vi "Frame Load Bmp and Img.vi"(8 "error in (no error)":errorcluster, 9 "PNG Path":path, 10 "File String":string, 11 "LF2R IDE in":refnum<class "LF2R IDE.lvclass">) -> (0 "error out":errorcluster, 3 "LF2R IDE out":refnum<class "LF2R IDE.lvclass">)   [LabVIEW 2018, in "LF2R IDE.lvlib" / "LF2R IDE.lvclass"]
uses:
  LF2R IDE.lvclass
  LF2R IDE.lvclass/LF2R IDE.ctl
  Frame Analizer/Data Parser.lvclass
  Image/Image Process.lvclass
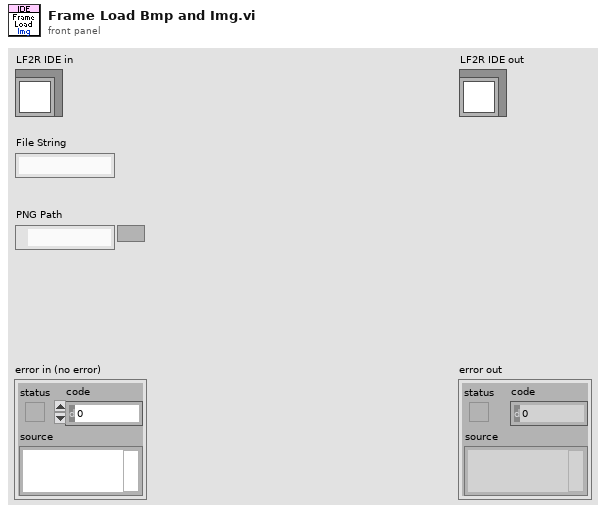
[diagram p1: front panel]
types:
  T1 = typedef "Data Parser.lvclass/Bmp data.ctl" = cluster{"File Data":T2[], "resized":string, "default_centerx":string, "default_centery":string}
  T2 = typedef "Data Parser.lvclass/Bmp File Data.ctl" = cluster{"Pic Start":i32, "Pic End":i32, "Json Path":string, "w":i32, "h":i32, "row":i32, "col":i32}
  T3 = typedef "Image Json Parser.lvclass/Img Json Data.ctl" = cluster{"frames":T4[], "meta":T5}
  T4 = typedef "Image Json Parser.lvclass/Img Json Frames.ctl" = cluster{"frame":cluster{"x":i32, "y":i32, "w":i32, "h":i32}, "rotated":bool, "trimmed":bool, "spriteSourceSize":cluster{"x":i32, "y":i32, "w":i32, "h":i32}, "sourceSize":cluster{"w":i32, "h":i32}}
  T5 = typedef "Image Json Parser.lvclass/Img Json Meta.ctl" = cluster{"app":string, "version":string, "image":string, "format":string, "size":cluster{"w":i32, "h":i32}, "scale":string}
  T6 = typedef "imagedata.ctl" = cluster{"image type":i32, "image depth":i32, "image":u8[], "mask":u8[], "colors":u32[], "Rectangle":cluster{"left":i16, "top":i16, "right":i16, "bottom":i16}}
  T7 = cluster{"image data":T6, "24-bit pixmap":u32[][]}
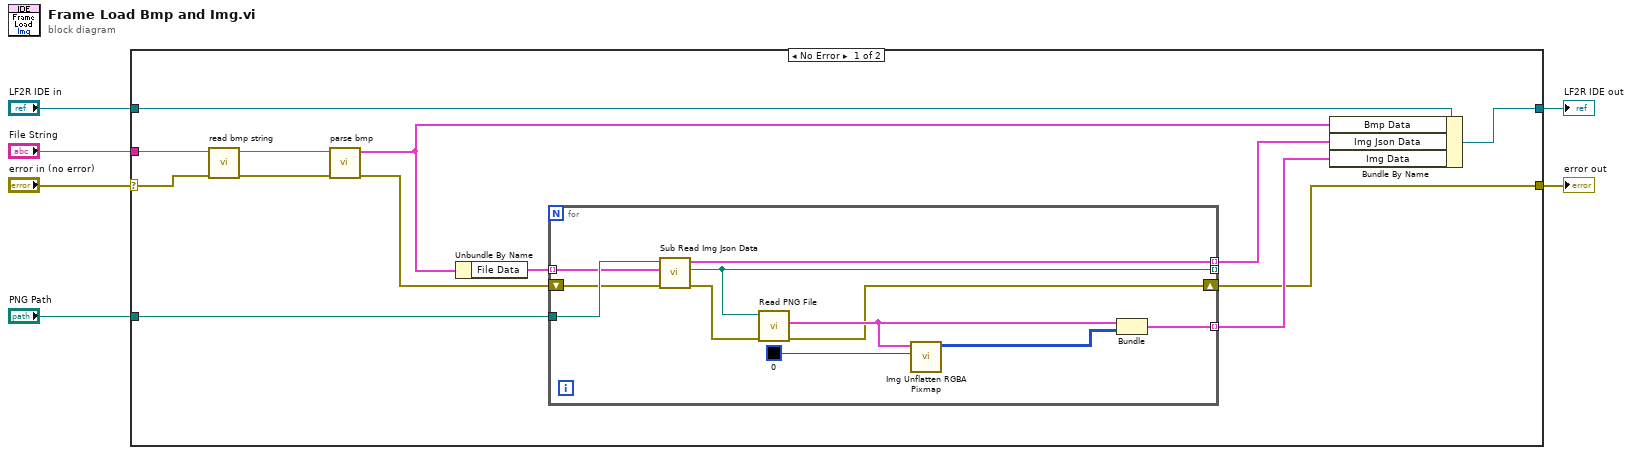
[diagram p0: block diagram]
diagram:
  n1 = case shown="No Error" "error in (no error)" {
    selector: "error in (no error)" -> [w15 w32]
    tunnel: [w7 w32] -> w5
    tunnel: [w14 w31] -> w3
    tunnel: "LF2R IDE in" -> [w19 w31]
    tunnel: "File String" -> [w16 _]
    tunnel: "PNG Path" -> [w13 _]
    frame No Error {
      n2 = call "read bmp string.vi"("error in"=w15, "file string"=w16) -> ("error out"=w17:errorcluster, "<bmp> string"=w18:string)  [unwired: 7 in, 1 out]
      n3 = call "parse bmp.vi"("error in (no error)"=w17, "<bmp> string"=w18) -> ("error out"=w9:errorcluster, "bmp data"=w12:T1)  [unwired: 8 in]
      n4 = Unbundle By Name(w12) -> ("File Data"=w11:T2[])
      n5 = for {
        tunnel: w13 -> [w30]
        tunnel: [w27] -> w10 mode=indexing
        shift-right: [w20] -> w7
        shift-left: w9 -> [w29]
        tunnel: w11 -> [w28] mode=indexing
        tunnel: [w26] -> _ mode=indexing
        tunnel: [w24] -> w8 mode=indexing
        n6 = call "Sub Read Img Json Data.vi"("error in"=w29, "File Data"=w28, "PNG Path"=w30) -> ("error out"=w25:errorcluster, "Image Path"=w26:path, "Json Data"=w27:T3)  [unwired: 6 in]
        n7 = call <vilib>:"Read PNG File.vi"("error in (no error)"=w25, "path to PNG file"=w26) -> ("error out"=w20:errorcluster, "image data"=w22:T6)  [unwired: 7 in, 1 out]
        n8 = call "Img Unflatten RGBA Pixmap.vi"("BG Color"=u32 0, "image data"=w22) -> ("24-bit pixmap"=w23:u32[][])  [unwired: 9 in]
        n9 = Bundle("image data"=w22, "24-bit pixmap"=w23) -> (w24:T7)  [unwired: 1 in]
      }
      n10 = Bundle By Name(cluster=w19, "Bmp Data"=w12, "Img Json Data"=w10, "Img Data"=w8) -> (w14:refnum<class "LF2R IDE.lvclass">)
    }
    frame Error {
    }
  }
  "error out" <- w5
  "LF2R IDE out" <- w3
